vi "USBL_UA TRACKER for boat.vi"() -> ()   [LabVIEW 2017]
uses:
  <vilib>/Analysis/2dsp.llb/Decimate (single shot, DBL).vi
  <vilib>/DAQmx/read.llb/DAQmx Read (Analog 1D Wfm NChan NSamp).vi
  <vilib>/Analysis/3filter.llb/FIR Filter (DBL).vi
  <vilib>/DAQmx/create/channels.llb/DAQmx Create Channel (AI-Voltage-Basic).vi
  <vilib>/DAQmx/configure/timing.llb/DAQmx Timing (Sample Clock).vi
  <vilib>/DAQmx/miscellaneous.llb/DAQmx Fill In Error Info.vi
  <vilib>/DAQmx/create/channels.llb/DAQmx Create Channel (CO-Pulse Generation-Frequency).vi
  <vilib>/DAQmx/configure/timing.llb/DAQmx Timing (Implicit).vi
  <vilib>/Analysis/NI_AALBase.lvlib
  <vilib>/Analysis/NI_AALPro.lvlib
  <vilib>/Analysis/NI_AAL_SigProc.lvlib
  <resource>/objmgr/daqmx.rc
panel:
  out "숫자형 8":dbl=5.0
  out "Target code":dbl[](array[numeric])
  out "ThresholdMargin":dbl=10.0
  out "MovingAvrParm":dbl[](array[numeric])
  out "Coefficient_bit1":dbl[](array[numeric])
  out "Coefficient_bit0":dbl[](array[numeric])
  out "Decimation rate":i32=12
  out "Carrier signal":dbl[](array[numeric])
  out "숫자형 7":dbl=7.0
  out "숫자형 6":dbl=7.0
  out "숫자형 5":dbl=7.0
  in  "Number of pulse":i32=1000
  in  "Output terminal":tag="/Dev1/PFI12"
  in  "Frequency(Hz)":dbl=1.0 format="%.6f"
  in  "Cycle share":dbl=0.5 format="%.6f"
  in  "Counter":tag="Dev1/ctr0"
  out "Detect":bool
  in  "User number":i32=12
  out "숫자형 4":dbl=5.0
  out "숫자형 3":dbl=7.0
  out "숫자형 2":dbl=7.0
  out "숫자형":dbl=7.0
  in  "Start frequency(Hz)":dbl format="%#_6p"
  in  "Stop frequency(Hz)":dbl=4000.0 format="%#_6p"
  in  "Symbol length(sec)":dbl=0.128 format="%#_6p"
  in  "Number of sample":i32=38400
  in  "Sampling freuqncy(Hz)":dbl=192000.0 format="%#_6p"
  in  "Physical channel":tag="Dev4/ai0:7" caption="Physical Channel"
  in  "Device":tag="Dev4"
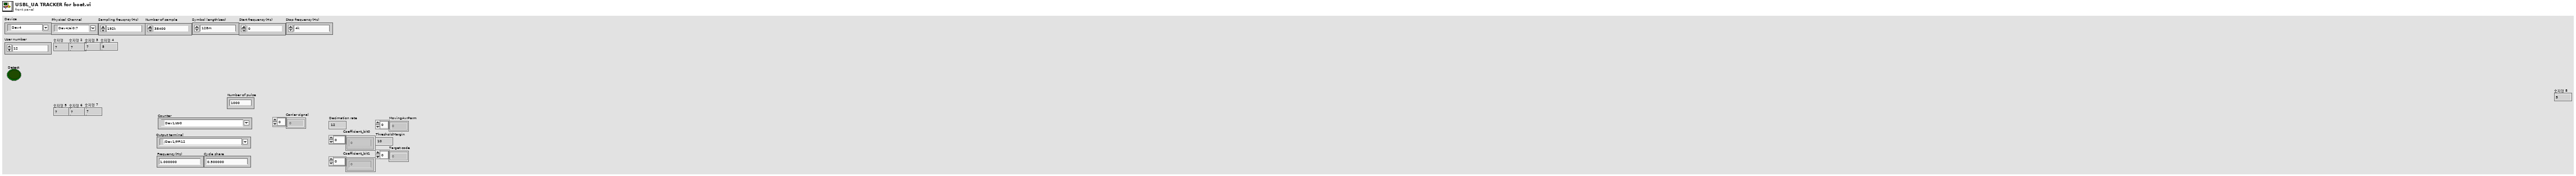
[diagram p1: front panel]
diagram:
  n1 = flat-sequence {
    tunnel: ["Number of sample"] -> w12
    tunnel: [w39] -> w11
    tunnel: ["Sampling freuqncy(Hz)"] -> w10
    tunnel: ["Physical channel"] -> w9
    tunnel: ["Device"] -> w8
    tunnel: [w35] -> w7
    tunnel: [w31] -> w6
    tunnel: [w30] -> w5
    tunnel: [w25] -> w4
    tunnel: [w21] -> w3
    tunnel: [w20] -> w2
    tunnel: [w13] -> w1
    tunnel: w12 -> [w59]
    tunnel: w11 -> [w58]
    tunnel: w10 -> [w57]
    tunnel: w9 -> [w56]
    tunnel: w8 -> [w55]
    tunnel: w7 -> [w54]
    tunnel: w6 -> [w53]
    tunnel: w5 -> [w52]
    tunnel: w4 -> [w49]
    tunnel: w3 -> [w47]
    tunnel: w2 -> [w46]
    tunnel: w1 -> [w43]
    frame #0 {
      w20 = 10.0 ("값")
      w22 = 160 ("차원 크기")
      w35 = 12 ("Divide by")
      w39 = 10123 items=["유한 샘플"=10178, "연속 샘플"=10123, "하드웨어 타이밍에 의한 단일 포인트"=12522] ("sample mode")
      # "Signal gen. (Counter)"
      # "Target code"
      # "EOF"
      # "SOF"
      # "Processing parameter"
      # "Freqeuncy 2"
      # "Freqeuncy 1"
      # "Symbol length"
      # "Moving average window size"
      # "Threshold Margin"
      # "DAQ device setting"
      # "Device"
      # "Physical channel"
      # "Sampling frequency"
      # "Sample mode"
      # "Number of samples per channel"
      n2 = To Double Precision Float(number=w35) -> (double precision float=w41:dbl)
      n3 = To Double Precision Float(number=w22) -> (double precision float=w24:dbl)
      n4 = Divide(x="Sampling freuqncy(Hz)", y=w41) -> (x/y=w29:dbl)
      n5 = Format Into String(format string="%04b" ("포맷 문자열"), "User number") -> (resulting string=w17:string)  [unwired: 2 in, 1 out]
      n6 = Reciprocal(x=w24) -> (1/x=w23:dbl)
      n7 = call "CodeConvert(SubVI).vi"("Code"=w17) -> ("Code_array"=w15:dbl[])
      n8 = Divide(x=30000.0, y="Sampling freuqncy(Hz)") -> (x/y=w33:dbl)
      n9 = Initialize Array(w23, w22) -> (w21:dbl[])
      "MovingAvrParm" <- w21
      n10 = call "ChirpSourceGen(SubVI).vi"("Frequency2(Hz)"="Stop frequency(Hz)", "Frequency1(Hz)"="Start frequency(Hz)", "Pulse length(sec)"="Symbol length(sec)", "Fs(Hz)"=w29) -> ("M.F. Tap(F2-1)"=w25:dbl[], "M.F. Tap(F1-2)"=w31:dbl[])  [unwired: 1 out]
      "Coefficient_bit0" <- w31
      "Coefficient_bit1" <- w25
      n11 = Insert Into Array(array=dbl[] [0.0, 1.0], new element #1=w15, new element #2=dbl[] [1.0, 0.0]) -> (w13:dbl[])  [unwired: 1 in]
      "Target code" <- w13
      n12 = call <vilib>:"Sine Wave.vi"("samples"="Number of sample", "amplitude"=5.0, "frequency"=w33) -> ("sine wave"=w30:dbl[])  [unwired: 2 in, 2 out]
      "Carrier signal" <- w30
      "Decimation rate" <- w35
      "ThresholdMargin" <- w20
    }
    frame #1 {
      n13 = flat-sequence {
        tunnel: w55 -> [w78]
        tunnel: [w79] -> w66
        tunnel: w56 -> [w77]
        tunnel: [w77] -> w65
        tunnel: w57 -> [w75]
        tunnel: [w75] -> w64
        tunnel: w59 -> [w74]
        tunnel: [w74] -> w63
        tunnel: w58 -> [w76]
        tunnel: [w76] -> w62
        tunnel: [w72] -> w61
        tunnel: [w73] -> w60
        tunnel: w54 -> [w73]
        tunnel: w53 -> [w72]
        tunnel: w52 -> [w71]
        tunnel: [w71] -> w51
        tunnel: [w70] -> w50
        tunnel: w49 -> [w70]
        tunnel: [w69] -> w48
        tunnel: w47 -> [w69]
        tunnel: w46 -> [w68]
        tunnel: [w68] -> w45
        tunnel: [w67] -> w44
        tunnel: w43 -> [w67]
        tunnel: w66 -> [w123]
        tunnel: w65 -> [w122]
        tunnel: w64 -> [w121]
        tunnel: w63 -> [w119]
        tunnel: w62 -> [w120]
        tunnel: w61 -> [w108]
        tunnel: w60 -> [w96]
        tunnel: w51 -> [w97]
        tunnel: w50 -> [w81]
        tunnel: w48 -> [w88]
        tunnel: w45 -> [w87]
        tunnel: w44 -> [w82]
        tunnel: [w430] -> w42
        tunnel: w42 -> [w523]
        frame #0 {
          n14 = call <vilib>:"DAQmx Reset Device.vi"("device in"=w78) -> ("error out"=w79:errorcluster)  [unwired: 1 in, 13 out]
        }
        frame #1 {
          w80 = dbl[] [-1.0, -1.0, -1.0, -1.0, -1.0, -1.0, -1.0, -1.0]
          w94 = "Proc1" ("이름(이름없음)")
          w95 = "Proc0" ("이름(이름없음)")
          w93 = dbl[][] []
          w109 = "SIG0" ("이름(이름없음)")
          w116 = waveform(dbl) {"t0"=timestamp(0 s since 1904-01-01), "dt"=1.0, "Y"=[]} ("Waveform")
          w99 = "SIG1" ("이름(이름없음)")
          # "Target code"
          # "[Post processing]  1. Queue get : Proc0, Proc1 / 2. Threshold estimation with moving average / 3. Peak and valley detection / 4. Demodulation"
          # "[Signal processing]\n1. Queue get : SIG0\n2. Data type converting : Waveform (DBL) --> Array (DBL)\n3. DDC (Digital to Digital Convering)\n  - DSB modulation : Multiply carrier signal (30kHz)\n  - Decimate : 192kHz sample rate --> 16kHz sample rate\n4. Cross-correlation with down-chirp (4k ~ 0Hz)\n5. Envelope detection (Hilbert transform) & square\n6. Queue put : Proc1"
          # "[Signal processing]\n1. Queue get : SIG0\n2. Data type converting : Waveform (DBL) --> Array (DBL)\n3. DDC (Digital to Digital Convering)\n  - DSB modulation : Multiply carrier signal (30kHz)\n  - Decimate : 192kHz sample rate --> 16kHz sample rate\n4. Cross-correlation with up-chirp (0 ~ 4kHz)\n5. Envelope detection (Hilbert transform) & square\n6. Queue put : Proc0"
          # "[Data Acquistion (ADC)]\n1. Device reset\n2. Creat channel\n3, Set sample clock\n  - Sampling frequency : 192kHz\n  - Number of sample (Chunk size) : 38400\n4. Start task\n5. Data read\n6. Queue put : SIG0, SIG1\n  - Queue data type : Waveform (DBL)"
          # "Moving average prameter based on FIR filter calculation"
          # "Coefficient for bit 1 : Down-chirp"
          # "Coefficient for bit 0 : Up-chirp"
          # "Decimation rate"
          # "Carrier signal"
          n15 = call-poly <vilib>:"DAQmx Create Virtual Channel.vi"("physical channels"=w122, "error in"=w123) -> ("task out"=w125:refnum<k21>, "error out"=w124:errorcluster)  [unwired: 7 in, 5 out]
          n16 = call-poly <vilib>:"DAQmx Timing.vi"("task/channels in"=w125, "sample mode"=w120, "samples per channel"=w119, "rate"=w121, "error in"=w124) -> ("task out"=w126:refnum<k21>, "error out"=w127:errorcluster)  [unwired: 2 in, 7 out]
          n17 = call <vilib>:"DAQmx Start Task.vi"("task/channels in"=w126, "error in"=w127) -> ("task out"=w128:refnum<k21>, "error out"=w129:errorcluster)  [unwired: 12 in]
          n18 = Build Array(w116, w116, w116, w116, w116, w116, w116, w116) -> (w98:waveform(dbl)[])
          n19 = Obtain Queue(name (unnamed)=w99, element data type=w98) -> (queue out=w118:refnum<queue>, error out=w117:errorcluster)  [unwired: 3 in, 1 out]
          n20 = Obtain Queue(name (unnamed)=w109, element data type=w98) -> (queue out=w115:refnum<queue>, error out=w114:errorcluster)  [unwired: 3 in, 1 out]
          n21 = while {
            tunnel: w128 -> [w429]
            tunnel: w129 -> [w428]
            tunnel: [w427] -> w132
            tunnel: [w426] -> w133
            tunnel: w119 -> [w425]
            tunnel: w118 -> [w424]
            tunnel: w117 -> [w423]
            tunnel: w115 -> [w422]
            tunnel: w114 -> [w421]
            i -> [w419]
            stop <- w418 stop-if-true
            n22 = call-poly <vilib>:"DAQmx Read.vi"("task/channels in"=w429, "number of samples per channel"=w425, "error in"=w428) -> ("task out"=w427:refnum<k21>, "data"=w420:waveform(dbl)[], "error out"=w426:errorcluster)  [unwired: 10 out]
            n23 = Enqueue Element(queue=w422, element=w420, error in (no error)=w421) -> ()  [unwired: 1 in, 3 out]
            n24 = Enqueue Element(queue=w424, element=w420, error in (no error)=w423) -> ()  [unwired: 1 in, 3 out]
            n25 = local read "Detect"() -> (w418:bool)
            "숫자형" <- w419
          }
          n26 = call <vilib>:"DAQmx Stop Task.vi"("task/channels in"=w132, "error in"=w133) -> ("task out"=w131:refnum<k21>, "error out"=w130:errorcluster)  [unwired: 12 out]
          n27 = call <vilib>:"DAQmx Clear Task.vi"("task in"=w131, "error in"=w130) -> ()  [unwired: 14 out]
          n28 = Obtain Queue(name (unnamed)=w95, element data type=w93) -> (queue out=w113:refnum<queue>, error out=w112:errorcluster)  [unwired: 3 in, 1 out]
          n29 = Obtain Queue(name (unnamed)=w109, element data type=w98) -> (queue out=w111:refnum<queue>, error out=w110:errorcluster)  [unwired: 3 in, 1 out]
          n30 = while {
            tunnel: w111 -> [w417]
            tunnel: w110 -> [w416]
            tunnel: w113 -> [w415]
            tunnel: w112 -> [w414]
            tunnel: [w413] -> w107
            tunnel: [w412] -> w106
            tunnel: w97 -> [w352]
            tunnel: w96 -> [w351]
            tunnel: w108 -> [w350]
            i -> [w348]
            stop <- w347 stop-if-true
            w362 = TRUE ("averaging")
            w411 = TRUE ("init/cont (init:F)")
            n31 = Dequeue Element(queue=w417, error in (no error)=w416) -> (queue out=w413:refnum<queue>, element=w353:waveform(dbl)[], error out=w412:errorcluster)  [unwired: 2 out]
            n32 = Index Array(array=w353) -> (element #1=w410:waveform(dbl), element #2=w409:waveform(dbl), element #3=w408:waveform(dbl), element #4=w407:waveform(dbl), element #5=w406:waveform(dbl), element #6=w405:waveform(dbl), element #7=w404:waveform(dbl), element #8=w403:waveform(dbl))  [unwired: 8 in]
            n33 = Unbundle By Name(w410) -> ("Y"=w402:dbl[])
            n34 = Unbundle By Name(w409) -> ("Y"=w401:dbl[])
            n35 = Unbundle By Name(w408) -> ("Y"=w400:dbl[])
            n36 = Unbundle By Name(w407) -> ("Y"=w399:dbl[])
            n37 = Unbundle By Name(w406) -> ("Y"=w398:dbl[])
            n38 = Unbundle By Name(w405) -> ("Y"=w397:dbl[])
            n39 = Unbundle By Name(w404) -> ("Y"=w396:dbl[])
            n40 = Unbundle By Name(w403) -> ("Y"=w395:dbl[])
            n41 = Multiply(x=w402, y=w352) -> (x*y=w377:dbl[])
            n42 = Multiply(x=w401, y=w352) -> (x*y=w376:dbl[])
            n43 = Multiply(x=w400, y=w352) -> (x*y=w375:dbl[])
            n44 = Multiply(x=w399, y=w352) -> (x*y=w374:dbl[])
            n45 = Multiply(x=w398, y=w352) -> (x*y=w373:dbl[])
            n46 = Multiply(x=w397, y=w352) -> (x*y=w372:dbl[])
            n47 = Multiply(x=w396, y=w352) -> (x*y=w371:dbl[])
            n48 = Multiply(x=w395, y=w352) -> (x*y=w370:dbl[])
            n49 = call-poly <vilib>:"Decimate (single shot).vi"("averaging"=w362, "decimating factor"=w351, "X"=w372) -> ("Decimated Array"=w365:dbl[])  [unwired: 7 in, 1 out]
            n50 = call-poly <vilib>:"Decimate (single shot).vi"("averaging"=w362, "decimating factor"=w351, "X"=w370) -> ("Decimated Array"=w363:dbl[])  [unwired: 7 in, 1 out]
            n51 = call-poly <vilib>:"Decimate (single shot).vi"("averaging"=w362, "decimating factor"=w351, "X"=w376) -> ("Decimated Array"=w369:dbl[])  [unwired: 7 in, 1 out]
            n52 = call-poly <vilib>:"Decimate (single shot).vi"("averaging"=w362, "decimating factor"=w351, "X"=w374) -> ("Decimated Array"=w367:dbl[])  [unwired: 7 in, 1 out]
            n53 = call-poly <vilib>:"Decimate (single shot).vi"("averaging"=w362, "decimating factor"=w351, "X"=w373) -> ("Decimated Array"=w366:dbl[])  [unwired: 7 in, 1 out]
            n54 = call-poly <vilib>:"Decimate (single shot).vi"("averaging"=w362, "decimating factor"=w351, "X"=w371) -> ("Decimated Array"=w364:dbl[])  [unwired: 7 in, 1 out]
            n55 = call-poly <vilib>:"Decimate (single shot).vi"("averaging"=w362, "decimating factor"=w351, "X"=w377) -> ("Decimated Array"=w378:dbl[])  [unwired: 7 in, 1 out]
            n56 = call-poly <vilib>:"Decimate (single shot).vi"("averaging"=w362, "decimating factor"=w351, "X"=w375) -> ("Decimated Array"=w368:dbl[])  [unwired: 7 in, 1 out]
            n57 = call-poly <vilib>:"FIR Filter.vi"("init/cont (init:F)"=w411, "FIR Coefficients"=w350, "X"=w378) -> ("Filtered X"=w394:dbl[])  [unwired: 1 in, 1 out]
            n58 = call-poly <vilib>:"FIR Filter.vi"("init/cont (init:F)"=w411, "FIR Coefficients"=w350, "X"=w369) -> ("Filtered X"=w393:dbl[])  [unwired: 1 in, 1 out]
            n59 = call-poly <vilib>:"FIR Filter.vi"("init/cont (init:F)"=w411, "FIR Coefficients"=w350, "X"=w368) -> ("Filtered X"=w392:dbl[])  [unwired: 1 in, 1 out]
            n60 = call-poly <vilib>:"FIR Filter.vi"("init/cont (init:F)"=w411, "FIR Coefficients"=w350, "X"=w367) -> ("Filtered X"=w391:dbl[])  [unwired: 1 in, 1 out]
            n61 = call-poly <vilib>:"FIR Filter.vi"("init/cont (init:F)"=w411, "FIR Coefficients"=w350, "X"=w366) -> ("Filtered X"=w390:dbl[])  [unwired: 1 in, 1 out]
            n62 = call-poly <vilib>:"FIR Filter.vi"("init/cont (init:F)"=w411, "FIR Coefficients"=w350, "X"=w365) -> ("Filtered X"=w389:dbl[])  [unwired: 1 in, 1 out]
            n63 = call-poly <vilib>:"FIR Filter.vi"("init/cont (init:F)"=w411, "FIR Coefficients"=w350, "X"=w364) -> ("Filtered X"=w388:dbl[])  [unwired: 1 in, 1 out]
            n64 = call-poly <vilib>:"FIR Filter.vi"("init/cont (init:F)"=w411, "FIR Coefficients"=w350, "X"=w363) -> ("Filtered X"=w387:dbl[])  [unwired: 1 in, 1 out]
            n65 = call "Envelope(SubVI).vi"("x"=w394) -> ("Y"=w386:dbl[])
            n66 = call "Envelope(SubVI).vi"("x"=w393) -> ("Y"=w385:dbl[])
            n67 = call "Envelope(SubVI).vi"("x"=w392) -> ("Y"=w384:dbl[])
            n68 = call "Envelope(SubVI).vi"("x"=w391) -> ("Y"=w383:dbl[])
            n69 = call "Envelope(SubVI).vi"("x"=w390) -> ("Y"=w382:dbl[])
            n70 = call "Envelope(SubVI).vi"("x"=w389) -> ("Y"=w381:dbl[])
            n71 = call "Envelope(SubVI).vi"("x"=w388) -> ("Y"=w380:dbl[])
            n72 = call "Envelope(SubVI).vi"("x"=w387) -> ("Y"=w379:dbl[])
            n73 = Square(x=w386) -> (x^2=w361:dbl[])
            n74 = Square(x=w385) -> (x^2=w360:dbl[])
            n75 = Square(x=w384) -> (x^2=w359:dbl[])
            n76 = Square(x=w383) -> (x^2=w358:dbl[])
            n77 = Square(x=w382) -> (x^2=w357:dbl[])
            n78 = Square(x=w381) -> (x^2=w356:dbl[])
            n79 = Square(x=w380) -> (x^2=w355:dbl[])
            n80 = Square(x=w379) -> (x^2=w354:dbl[])
            n81 = local read "Detect"() -> (w347:bool)
            n82 = Build Array(w361, w360, w359, w358, w357, w356, w355, w354) -> (w349:dbl[][])
            n83 = Enqueue Element(queue=w415, element=w349, error in (no error)=w414) -> ()  [unwired: 1 in, 3 out]
            "숫자형 2" <- w348
          }
          n84 = Release Queue(queue=w107, error in (no error)=w106) -> ()  [unwired: 1 in, 3 out]
          n85 = Obtain Queue(name (unnamed)=w94, element data type=w93) -> (queue out=w105:refnum<queue>, error out=w104:errorcluster)  [unwired: 3 in, 1 out]
          n86 = Obtain Queue(name (unnamed)=w99, element data type=w98) -> (queue out=w103:refnum<queue>, error out=w102:errorcluster)  [unwired: 3 in, 1 out]
          n87 = while {
            tunnel: w103 -> [w346]
            tunnel: w102 -> [w345]
            tunnel: w105 -> [w344]
            tunnel: w104 -> [w343]
            tunnel: [w342] -> w101
            tunnel: [w341] -> w100
            tunnel: w97 -> [w281]
            tunnel: w96 -> [w280]
            tunnel: w81 -> [w279]
            i -> [w277]
            stop <- w276 stop-if-true
            w291 = TRUE ("averaging")
            w340 = TRUE ("init/cont (init:F)")
            n88 = Dequeue Element(queue=w346, error in (no error)=w345) -> (queue out=w342:refnum<queue>, element=w282:waveform(dbl)[], error out=w341:errorcluster)  [unwired: 2 out]
            n89 = Index Array(array=w282) -> (element #1=w339:waveform(dbl), element #2=w338:waveform(dbl), element #3=w337:waveform(dbl), element #4=w336:waveform(dbl), element #5=w335:waveform(dbl), element #6=w334:waveform(dbl), element #7=w333:waveform(dbl), element #8=w332:waveform(dbl))  [unwired: 8 in]
            n90 = Unbundle By Name(w339) -> ("Y"=w331:dbl[])
            n91 = Unbundle By Name(w338) -> ("Y"=w330:dbl[])
            n92 = Unbundle By Name(w337) -> ("Y"=w329:dbl[])
            n93 = Unbundle By Name(w336) -> ("Y"=w328:dbl[])
            n94 = Unbundle By Name(w335) -> ("Y"=w327:dbl[])
            n95 = Unbundle By Name(w334) -> ("Y"=w326:dbl[])
            n96 = Unbundle By Name(w333) -> ("Y"=w325:dbl[])
            n97 = Unbundle By Name(w332) -> ("Y"=w324:dbl[])
            n98 = Multiply(x=w331, y=w281) -> (x*y=w306:dbl[])
            n99 = Multiply(x=w330, y=w281) -> (x*y=w305:dbl[])
            n100 = Multiply(x=w329, y=w281) -> (x*y=w304:dbl[])
            n101 = Multiply(x=w328, y=w281) -> (x*y=w303:dbl[])
            n102 = Multiply(x=w327, y=w281) -> (x*y=w302:dbl[])
            n103 = Multiply(x=w326, y=w281) -> (x*y=w301:dbl[])
            n104 = Multiply(x=w325, y=w281) -> (x*y=w300:dbl[])
            n105 = Multiply(x=w324, y=w281) -> (x*y=w299:dbl[])
            n106 = call-poly <vilib>:"Decimate (single shot).vi"("averaging"=w291, "decimating factor"=w280, "X"=w301) -> ("Decimated Array"=w294:dbl[])  [unwired: 7 in, 1 out]
            n107 = call-poly <vilib>:"Decimate (single shot).vi"("averaging"=w291, "decimating factor"=w280, "X"=w299) -> ("Decimated Array"=w292:dbl[])  [unwired: 7 in, 1 out]
            n108 = call-poly <vilib>:"Decimate (single shot).vi"("averaging"=w291, "decimating factor"=w280, "X"=w305) -> ("Decimated Array"=w298:dbl[])  [unwired: 7 in, 1 out]
            n109 = call-poly <vilib>:"Decimate (single shot).vi"("averaging"=w291, "decimating factor"=w280, "X"=w303) -> ("Decimated Array"=w296:dbl[])  [unwired: 7 in, 1 out]
            n110 = call-poly <vilib>:"Decimate (single shot).vi"("averaging"=w291, "decimating factor"=w280, "X"=w302) -> ("Decimated Array"=w295:dbl[])  [unwired: 7 in, 1 out]
            n111 = call-poly <vilib>:"Decimate (single shot).vi"("averaging"=w291, "decimating factor"=w280, "X"=w300) -> ("Decimated Array"=w293:dbl[])  [unwired: 7 in, 1 out]
            n112 = call-poly <vilib>:"Decimate (single shot).vi"("averaging"=w291, "decimating factor"=w280, "X"=w306) -> ("Decimated Array"=w307:dbl[])  [unwired: 7 in, 1 out]
            n113 = call-poly <vilib>:"Decimate (single shot).vi"("averaging"=w291, "decimating factor"=w280, "X"=w304) -> ("Decimated Array"=w297:dbl[])  [unwired: 7 in, 1 out]
            n114 = call-poly <vilib>:"FIR Filter.vi"("init/cont (init:F)"=w340, "FIR Coefficients"=w279, "X"=w307) -> ("Filtered X"=w323:dbl[])  [unwired: 1 in, 1 out]
            n115 = call-poly <vilib>:"FIR Filter.vi"("init/cont (init:F)"=w340, "FIR Coefficients"=w279, "X"=w298) -> ("Filtered X"=w322:dbl[])  [unwired: 1 in, 1 out]
            n116 = call-poly <vilib>:"FIR Filter.vi"("init/cont (init:F)"=w340, "FIR Coefficients"=w279, "X"=w297) -> ("Filtered X"=w321:dbl[])  [unwired: 1 in, 1 out]
            n117 = call-poly <vilib>:"FIR Filter.vi"("init/cont (init:F)"=w340, "FIR Coefficients"=w279, "X"=w296) -> ("Filtered X"=w320:dbl[])  [unwired: 1 in, 1 out]
            n118 = call-poly <vilib>:"FIR Filter.vi"("init/cont (init:F)"=w340, "FIR Coefficients"=w279, "X"=w295) -> ("Filtered X"=w319:dbl[])  [unwired: 1 in, 1 out]
            n119 = call-poly <vilib>:"FIR Filter.vi"("init/cont (init:F)"=w340, "FIR Coefficients"=w279, "X"=w294) -> ("Filtered X"=w318:dbl[])  [unwired: 1 in, 1 out]
            n120 = call-poly <vilib>:"FIR Filter.vi"("init/cont (init:F)"=w340, "FIR Coefficients"=w279, "X"=w293) -> ("Filtered X"=w317:dbl[])  [unwired: 1 in, 1 out]
            n121 = call-poly <vilib>:"FIR Filter.vi"("init/cont (init:F)"=w340, "FIR Coefficients"=w279, "X"=w292) -> ("Filtered X"=w316:dbl[])  [unwired: 1 in, 1 out]
            n122 = call "Envelope(SubVI).vi"("x"=w323) -> ("Y"=w315:dbl[])
            n123 = call "Envelope(SubVI).vi"("x"=w322) -> ("Y"=w314:dbl[])
            n124 = call "Envelope(SubVI).vi"("x"=w321) -> ("Y"=w313:dbl[])
            n125 = call "Envelope(SubVI).vi"("x"=w320) -> ("Y"=w312:dbl[])
            n126 = call "Envelope(SubVI).vi"("x"=w319) -> ("Y"=w311:dbl[])
            n127 = call "Envelope(SubVI).vi"("x"=w318) -> ("Y"=w310:dbl[])
            n128 = call "Envelope(SubVI).vi"("x"=w317) -> ("Y"=w309:dbl[])
            n129 = call "Envelope(SubVI).vi"("x"=w316) -> ("Y"=w308:dbl[])
            n130 = Square(x=w315) -> (x^2=w290:dbl[])
            n131 = Square(x=w314) -> (x^2=w289:dbl[])
            n132 = Square(x=w313) -> (x^2=w288:dbl[])
            n133 = Square(x=w312) -> (x^2=w287:dbl[])
            n134 = Square(x=w311) -> (x^2=w286:dbl[])
            n135 = Square(x=w310) -> (x^2=w285:dbl[])
            n136 = Square(x=w309) -> (x^2=w284:dbl[])
            n137 = Square(x=w308) -> (x^2=w283:dbl[])
            n138 = local read "Detect"() -> (w276:bool)
            n139 = Build Array(w290, w289, w288, w287, w286, w285, w284, w283) -> (w278:dbl[][])
            n140 = Enqueue Element(queue=w344, element=w278, error in (no error)=w343) -> ()  [unwired: 1 in, 3 out]
            "숫자형 3" <- w277
          }
          n141 = Release Queue(queue=w101, error in (no error)=w100) -> ()  [unwired: 1 in, 3 out]
          n142 = Obtain Queue(name (unnamed)=w95, element data type=w93) -> (queue out=w92:refnum<queue>, error out=w91:errorcluster)  [unwired: 3 in, 1 out]
          n143 = Obtain Queue(name (unnamed)=w94, element data type=w93) -> (queue out=w90:refnum<queue>, error out=w89:errorcluster)  [unwired: 3 in, 1 out]
          n144 = while {
            tunnel: w92 -> [w275]
            tunnel: w91 -> [w274]
            tunnel: w90 -> [w273]
            tunnel: w89 -> [w272]
            tunnel: w88 -> [w270]
            tunnel: w87 -> [w234]
            tunnel: [w182] -> w86
            tunnel: [w181] -> w85
            tunnel: [w180] -> w84
            tunnel: [w179] -> w83
            tunnel: w82 -> [w178]
            shift-right: [w141] -> _
            shift-left: w80 -> [w157]
            shift-right: [w140] -> _
            shift-left: w80 -> [w156]
            shift-right: [w139] -> _
            shift-left: w80 -> [w155]
            shift-right: [w138] -> _
            shift-left: w80 -> [w154]
            shift-right: [w137] -> _
            shift-left: w80 -> [w153]
            shift-right: [w136] -> _
            shift-left: w80 -> [w152]
            shift-right: [w135] -> _
            shift-left: w80 -> [w151]
            shift-right: [w134] -> _
            shift-left: w80 -> [w150]
            i -> [w166]
            stop <- w167 stop-if-true
            w259 = enum32{"Peaks", "Valleys"}."Valleys" ("peaks/valleys")
            w260 = enum32{"Peaks", "Valleys"}."Peaks" ("peaks/valleys")
            w258 = 5 ("width")
            w269 = TRUE ("init/cont (init:F)")
            n145 = Dequeue Element(queue=w275, error in (no error)=w274) -> (queue out=w182:refnum<queue>, element=w216:dbl[][], error out=w181:errorcluster)  [unwired: 2 out]
            n146 = Dequeue Element(queue=w273, error in (no error)=w272) -> (queue out=w180:refnum<queue>, element=w215:dbl[][], error out=w179:errorcluster)  [unwired: 2 out]
            n147 = Subtract(x=w216, y=w215) -> (x-y=w271:dbl[][])
            n148 = Index Array(array=w271) -> (element #1=w257:dbl[], element #2=w256:dbl[], element #3=w255:dbl[], element #4=w254:dbl[], element #5=w253:dbl[], element #6=w252:dbl[], element #7=w251:dbl[], element #8=w219:dbl[])  [unwired: 16 in]
            n149 = call-poly <vilib>:"FIR Filter.vi"("init/cont (init:F)"=w269, "FIR Coefficients"=w270, "X"=w257) -> ("Filtered X"=w268:dbl[])  [unwired: 1 in, 1 out]
            n150 = call-poly <vilib>:"FIR Filter.vi"("init/cont (init:F)"=w269, "FIR Coefficients"=w270, "X"=w256) -> ("Filtered X"=w267:dbl[])  [unwired: 1 in, 1 out]
            n151 = call-poly <vilib>:"FIR Filter.vi"("init/cont (init:F)"=w269, "FIR Coefficients"=w270, "X"=w255) -> ("Filtered X"=w266:dbl[])  [unwired: 1 in, 1 out]
            n152 = call-poly <vilib>:"FIR Filter.vi"("init/cont (init:F)"=w269, "FIR Coefficients"=w270, "X"=w254) -> ("Filtered X"=w265:dbl[])  [unwired: 1 in, 1 out]
            n153 = call-poly <vilib>:"FIR Filter.vi"("init/cont (init:F)"=w269, "FIR Coefficients"=w270, "X"=w253) -> ("Filtered X"=w264:dbl[])  [unwired: 1 in, 1 out]
            n154 = call-poly <vilib>:"FIR Filter.vi"("init/cont (init:F)"=w269, "FIR Coefficients"=w270, "X"=w252) -> ("Filtered X"=w263:dbl[])  [unwired: 1 in, 1 out]
            n155 = call-poly <vilib>:"FIR Filter.vi"("init/cont (init:F)"=w269, "FIR Coefficients"=w270, "X"=w251) -> ("Filtered X"=w262:dbl[])  [unwired: 1 in, 1 out]
            n156 = call-poly <vilib>:"FIR Filter.vi"("init/cont (init:F)"=w269, "FIR Coefficients"=w270, "X"=w219) -> ("Filtered X"=w261:dbl[])  [unwired: 1 in, 1 out]
            n157 = Array Max & Min(array=w268) -> (max value=w250:dbl, min value=w249:dbl)  [unwired: 2 out]
            n158 = Array Max & Min(array=w267) -> (max value=w248:dbl, min value=w247:dbl)  [unwired: 2 out]
            n159 = Array Max & Min(array=w266) -> (max value=w246:dbl, min value=w245:dbl)  [unwired: 2 out]
            n160 = Array Max & Min(array=w265) -> (max value=w244:dbl, min value=w243:dbl)  [unwired: 2 out]
            n161 = Array Max & Min(array=w264) -> (max value=w242:dbl, min value=w241:dbl)  [unwired: 2 out]
            n162 = Array Max & Min(array=w263) -> (max value=w240:dbl, min value=w239:dbl)  [unwired: 2 out]
            n163 = Array Max & Min(array=w262) -> (max value=w238:dbl, min value=w237:dbl)  [unwired: 2 out]
            n164 = Array Max & Min(array=w261) -> (max value=w236:dbl, min value=w235:dbl)  [unwired: 2 out]
            n165 = call "ThresholdEstimation(SubVI).vi"("Margin"=w234, "최소값"=w247, "최대값"=w248) -> ("N.Th"=w221:dbl, "P.Th"=w232:dbl)
            n166 = call "ThresholdEstimation(SubVI).vi"("Margin"=w234, "최소값"=w245, "최대값"=w246) -> ("N.Th"=w222:dbl, "P.Th"=w231:dbl)
            n167 = call "ThresholdEstimation(SubVI).vi"("Margin"=w234, "최소값"=w243, "최대값"=w244) -> ("N.Th"=w223:dbl, "P.Th"=w230:dbl)
            n168 = call "ThresholdEstimation(SubVI).vi"("Margin"=w234, "최소값"=w241, "최대값"=w242) -> ("N.Th"=w224:dbl, "P.Th"=w229:dbl)
            n169 = call "ThresholdEstimation(SubVI).vi"("Margin"=w234, "최소값"=w249, "최대값"=w250) -> ("N.Th"=w220:dbl, "P.Th"=w233:dbl)
            n170 = call "ThresholdEstimation(SubVI).vi"("Margin"=w234, "최소값"=w239, "최대값"=w240) -> ("N.Th"=w225:dbl, "P.Th"=w228:dbl)
            n171 = call "ThresholdEstimation(SubVI).vi"("Margin"=w234, "최소값"=w237, "최대값"=w238) -> ("N.Th"=w226:dbl, "P.Th"=w227:dbl)
            n172 = call "ThresholdEstimation(SubVI).vi"("Margin"=w234, "최소값"=w235, "최대값"=w236) -> ("N.Th"=w218:dbl, "P.Th"=w217:dbl)
            n173 = call <vilib>:"Peak Detector.vi"("peaks/valleys"=w260, "width"=w258, "threshold"=w233, "X"=w257) -> ("Locations"=w191:dbl[], "# found"=w207:i32)  [unwired: 3 in, 3 out]
            n174 = call <vilib>:"Peak Detector.vi"("peaks/valleys"=w260, "width"=w258, "threshold"=w232, "X"=w256) -> ("Locations"=w192:dbl[], "# found"=w208:i32)  [unwired: 3 in, 3 out]
            n175 = call <vilib>:"Peak Detector.vi"("peaks/valleys"=w260, "width"=w258, "threshold"=w231, "X"=w255) -> ("Locations"=w193:dbl[], "# found"=w209:i32)  [unwired: 3 in, 3 out]
            n176 = call <vilib>:"Peak Detector.vi"("peaks/valleys"=w260, "width"=w258, "threshold"=w230, "X"=w254) -> ("Locations"=w194:dbl[], "# found"=w210:i32)  [unwired: 3 in, 3 out]
            n177 = call <vilib>:"Peak Detector.vi"("peaks/valleys"=w260, "width"=w258, "threshold"=w229, "X"=w253) -> ("Locations"=w195:dbl[], "# found"=w211:i32)  [unwired: 3 in, 3 out]
            n178 = call <vilib>:"Peak Detector.vi"("peaks/valleys"=w260, "width"=w258, "threshold"=w228, "X"=w252) -> ("Locations"=w196:dbl[], "# found"=w212:i32)  [unwired: 3 in, 3 out]
            n179 = call <vilib>:"Peak Detector.vi"("peaks/valleys"=w260, "width"=w258, "threshold"=w227, "X"=w251) -> ("Locations"=w197:dbl[], "# found"=w213:i32)  [unwired: 3 in, 3 out]
            n180 = call <vilib>:"Peak Detector.vi"("peaks/valleys"=w260, "width"=w258, "threshold"=w217, "X"=w219) -> ("Locations"=w198:dbl[], "# found"=w214:i32)  [unwired: 3 in, 3 out]
            n181 = call <vilib>:"Peak Detector.vi"("peaks/valleys"=w259, "width"=w258, "threshold"=w220, "X"=w257) -> ("Locations"=w190:dbl[], "# found"=w206:i32)  [unwired: 3 in, 3 out]
            n182 = call <vilib>:"Peak Detector.vi"("peaks/valleys"=w259, "width"=w258, "threshold"=w221, "X"=w256) -> ("Locations"=w189:dbl[], "# found"=w205:i32)  [unwired: 3 in, 3 out]
            n183 = call <vilib>:"Peak Detector.vi"("peaks/valleys"=w259, "width"=w258, "threshold"=w222, "X"=w255) -> ("Locations"=w188:dbl[], "# found"=w204:i32)  [unwired: 3 in, 3 out]
            n184 = call <vilib>:"Peak Detector.vi"("peaks/valleys"=w259, "width"=w258, "threshold"=w223, "X"=w254) -> ("Locations"=w187:dbl[], "# found"=w203:i32)  [unwired: 3 in, 3 out]
            n185 = call <vilib>:"Peak Detector.vi"("peaks/valleys"=w259, "width"=w258, "threshold"=w224, "X"=w253) -> ("Locations"=w186:dbl[], "# found"=w202:i32)  [unwired: 3 in, 3 out]
            n186 = call <vilib>:"Peak Detector.vi"("peaks/valleys"=w259, "width"=w258, "threshold"=w225, "X"=w252) -> ("Locations"=w185:dbl[], "# found"=w201:i32)  [unwired: 3 in, 3 out]
            n187 = call <vilib>:"Peak Detector.vi"("peaks/valleys"=w259, "width"=w258, "threshold"=w226, "X"=w251) -> ("Locations"=w184:dbl[], "# found"=w200:i32)  [unwired: 3 in, 3 out]
            n188 = call <vilib>:"Peak Detector.vi"("peaks/valleys"=w259, "width"=w258, "threshold"=w218, "X"=w219) -> ("Locations"=w183:dbl[], "# found"=w199:i32)  [unwired: 3 in, 3 out]
            n189 = call "Decision(SubVI).vi"("L_ind0"=w207, "L_ind1"=w206, "Peak_ind0"=w191, "Peak_ind1"=w190) -> ("L_sum"=w149:i32, "Bits"=w165:dbl[])  [unwired: 2 in]
            n190 = call "Decision(SubVI).vi"("L_ind0"=w208, "L_ind1"=w205, "Peak_ind0"=w192, "Peak_ind1"=w189) -> ("L_sum"=w148:i32, "Bits"=w164:dbl[])  [unwired: 2 in]
            n191 = call "Decision(SubVI).vi"("L_ind0"=w209, "L_ind1"=w204, "Peak_ind0"=w193, "Peak_ind1"=w188) -> ("L_sum"=w147:i32, "Bits"=w163:dbl[])  [unwired: 2 in]
            n192 = call "Decision(SubVI).vi"("L_ind0"=w210, "L_ind1"=w203, "Peak_ind0"=w194, "Peak_ind1"=w187) -> ("L_sum"=w146:i32, "Bits"=w162:dbl[])  [unwired: 2 in]
            n193 = call "Decision(SubVI).vi"("L_ind0"=w211, "L_ind1"=w202, "Peak_ind0"=w195, "Peak_ind1"=w186) -> ("L_sum"=w145:i32, "Bits"=w161:dbl[])  [unwired: 2 in]
            n194 = call "Decision(SubVI).vi"("L_ind0"=w212, "L_ind1"=w201, "Peak_ind0"=w196, "Peak_ind1"=w185) -> ("L_sum"=w144:i32, "Bits"=w160:dbl[])  [unwired: 2 in]
            n195 = call "Decision(SubVI).vi"("L_ind0"=w213, "L_ind1"=w200, "Peak_ind0"=w197, "Peak_ind1"=w184) -> ("L_sum"=w143:i32, "Bits"=w159:dbl[])  [unwired: 2 in]
            n196 = call "Decision(SubVI).vi"("L_ind0"=w214, "L_ind1"=w199, "Peak_ind0"=w198, "Peak_ind1"=w183) -> ("L_sum"=w142:i32, "Bits"=w158:dbl[])  [unwired: 2 in]
            n197 = call "DataBuffer(SubVI).vi"("Bits"=w165, "Buffer"=w157) -> ("Data"=w141:dbl[])  [unwired: 2 in]
            n198 = call "DataBuffer(SubVI).vi"("Bits"=w164, "Buffer"=w156) -> ("Data"=w140:dbl[])  [unwired: 2 in]
            n199 = call "DataBuffer(SubVI).vi"("Bits"=w163, "Buffer"=w155) -> ("Data"=w139:dbl[])  [unwired: 2 in]
            n200 = call "DataBuffer(SubVI).vi"("Bits"=w162, "Buffer"=w154) -> ("Data"=w138:dbl[])  [unwired: 2 in]
            n201 = call "DataBuffer(SubVI).vi"("Bits"=w161, "Buffer"=w153) -> ("Data"=w137:dbl[])  [unwired: 2 in]
            n202 = call "DataBuffer(SubVI).vi"("Bits"=w160, "Buffer"=w152) -> ("Data"=w136:dbl[])  [unwired: 2 in]
            n203 = call "DataBuffer(SubVI).vi"("Bits"=w159, "Buffer"=w151) -> ("Data"=w135:dbl[])  [unwired: 2 in]
            n204 = call "DataBuffer(SubVI).vi"("Bits"=w158, "Buffer"=w150) -> ("Data"=w134:dbl[])  [unwired: 2 in]
            n205 = call "CodeDetection(SubVI).vi"("Code"=w178, "Buff"=w141, "L_sum"=w149) -> ("detect"=w177:bool)
            n206 = call "CodeDetection(SubVI).vi"("Code"=w178, "Buff"=w140, "L_sum"=w148) -> ("detect"=w176:bool)
            n207 = call "CodeDetection(SubVI).vi"("Code"=w178, "Buff"=w139, "L_sum"=w147) -> ("detect"=w175:bool)
            n208 = call "CodeDetection(SubVI).vi"("Code"=w178, "Buff"=w138, "L_sum"=w146) -> ("detect"=w174:bool)
            n209 = call "CodeDetection(SubVI).vi"("Code"=w178, "Buff"=w137, "L_sum"=w145) -> ("detect"=w173:bool)
            n210 = call "CodeDetection(SubVI).vi"("Code"=w178, "Buff"=w136, "L_sum"=w144) -> ("detect"=w172:bool)
            n211 = call "CodeDetection(SubVI).vi"("Code"=w178, "Buff"=w135, "L_sum"=w143) -> ("detect"=w171:bool)
            n212 = call "CodeDetection(SubVI).vi"("Code"=w178, "Buff"=w134, "L_sum"=w142) -> ("detect"=w170:bool)
            n213 = Build Array(w177, w176, w175, w174, w173, w172, w171, w170) -> (w169:bool[])
            n214 = Boolean Array To Number(Boolean array=w169) -> (number=w168:u32)
            n215 = Greater Than 0?(x=w168) -> (x > 0?=w167:bool)
            "Detect" <- w167
            "숫자형 4" <- w166
          }
          n216 = Release Queue(queue=w86, error in (no error)=w85) -> ()  [unwired: 1 in, 3 out]
          n217 = Release Queue(queue=w84, error in (no error)=w83) -> ()  [unwired: 1 in, 3 out]
        }
        frame #2 {
          n218 = local read "Device"() -> (w431:tag)
          n219 = call <vilib>:"DAQmx Reset Device.vi"("device in"=w431) -> ("error out"=w430:errorcluster)  [unwired: 1 in, 13 out]
        }
        frame #3 {
          w436 = dbl[] [-1.0, -1.0, -1.0, -1.0, -1.0, -1.0, -1.0, -1.0]
          w450 = dbl[][] []
          w466 = waveform(dbl) {"t0"=timestamp(0 s since 1904-01-01), "dt"=1.0, "Y"=[]} ("Waveform")
          w439 = "Proc1" ("이름(이름없음)")
          w438 = "Proc0" ("이름(이름없음)")
          w437 = dbl[][] []
          w489 = "SIG0" ("이름(이름없음)")
          w496 = waveform(dbl) {"t0"=timestamp(0 s since 1904-01-01), "dt"=1.0, "Y"=[]} ("Waveform")
          w480 = "SIG1" ("이름(이름없음)")
          w512 = 10123 items=["유한 샘플"=10178, "연속 샘플"=10123, "하드웨어 타이밍에 의한 단일 포인트"=12522] ("sample mode")
          w516 = 10178 items=["유한 샘플"=10178, "연속 샘플"=10123, "하드웨어 타이밍에 의한 단일 포인트"=12522] ("sample mode")
          # "[Post processing]  1. Queue get : Proc0, Proc1 / 2. Threshold estimation with moving average / 3. Peak and valley detection / 4. Demodulation"
          # "[Rx.time]\nTravel time (1km) : 670ms * 2\nDown-link : 210ms\nUp-link : 1024ms\nTotal : Rx.time > 2574ms"
          # "Local variable"
          # "Queue clear"
          # "[Data Acquistion (ADC)]"
          # "Signal generation (Counter) / delaty time : 200ms"
          # "[Signal processing]\n1. Queue get : SIG0\n2. Data type converting : Waveform (DBL) --> Array (DBL)\n3. DDC (Digital to Digital Convering)\n  - DSB modulation : Multiply carrier signal (30kHz)\n  - Decimate : 192kHz sample rate --> 16kHz sample rate\n4. Cross-correlation with down-chirp (4k ~ 0Hz)\n5. Envelope detection (Hilbert transform) & square\n6. Queue put : Proc1"
          # "[Signal processing]\n1. Queue get : SIG0\n2. Data type converting : Waveform (DBL) --> Array (DBL)\n3. DDC (Digital to Digital Convering)\n  - DSB modulation : Multiply carrier signal (30kHz)\n  - Decimate : 192kHz sample rate --> 16kHz sample rate\n4. Cross-correlation with up-chirp (0 ~ 4kHz)\n5. Envelope detection (Hilbert transform) & square\n6. Queue put : Proc0"
          # "[Data Acquistion (ADC)]\n1. Device reset\n2. Creat channel\n3, Set sample clock\n  - Sampling frequency : 192kHz\n  - Number of sample (Chunk size) : 38400\n4. Start task\n5. Data read\n6. Queue put : SIG0, SIG1\n  - Queue data type : Waveform (DBL)"
          n220 = local read "Number of pulse"() -> (w517:i32)
          n221 = local read "Output terminal"() -> (w520:tag)
          n222 = local read "Sampling freuqncy(Hz)"() -> (w448:dbl)
          n223 = local read "Physical channel"() -> (w514:tag)
          n224 = local read "Frequency(Hz)"() -> (w525:dbl)
          n225 = Build Array(w466, w466, w466, w466, w466, w466, w466, w466) -> (w465:waveform(dbl)[])
          n226 = local read "Cycle share"() -> (w524:dbl)
          n227 = local read "Number of sample"() -> (w447:i32)
          n228 = local read "Counter"() -> (w526:tag)
          n229 = Obtain Queue(name (unnamed)="SIG1" ("이름(이름없음)"), element data type=w465) -> (queue out=w462:refnum<queue>, error out=w461:errorcluster)  [unwired: 3 in, 1 out]
          n230 = Obtain Queue(name (unnamed)="Proc1" ("이름(이름없음)"), element data type=w450) -> (queue out=w454:refnum<queue>, error out=w453:errorcluster)  [unwired: 3 in, 1 out]
          n231 = Obtain Queue(name (unnamed)="SIG0" ("이름(이름없음)"), element data type=w465) -> (queue out=w472:refnum<queue>, error out=w471:errorcluster)  [unwired: 3 in, 1 out]
          n232 = Obtain Queue(name (unnamed)="Proc0" ("이름(이름없음)"), element data type=w450) -> (queue out=w460:refnum<queue>, error out=w459:errorcluster)  [unwired: 3 in, 1 out]
          n233 = call-poly <vilib>:"DAQmx Create Virtual Channel.vi"("frequency"=w525, "duty cycle"=w524, "counter"=w526, "error in"=w523) -> ("task out"=w522:refnum<k21>, "error out"=w521:errorcluster)  [unwired: 10 in]
          n234 = call-poly <vilib>:"DAQmx Create Virtual Channel.vi"("physical channels"=w514) -> ("task out"=w513:refnum<k21>, "error out"=w515:errorcluster)  [unwired: 8 in, 5 out]
          n235 = Flush Queue(queue=w472, error in (no error)=w471) -> (queue out=w470:refnum<queue>, error out=w469:errorcluster)  [unwired: 1 out]
          n236 = Flush Queue(queue=w462, error in (no error)=w461) -> (queue out=w464:refnum<queue>, error out=w463:errorcluster)  [unwired: 1 out]
          n237 = Flush Queue(queue=w460, error in (no error)=w459) -> (queue out=w458:refnum<queue>, error out=w457:errorcluster)  [unwired: 1 out]
          n238 = Flush Queue(queue=w454, error in (no error)=w453) -> (queue out=w456:refnum<queue>, error out=w455:errorcluster)  [unwired: 1 out]
          n239 = property class="DAQmx 채널"(reference=w522, error in=w521, "CO.Pulse.Term"=w520) -> (reference out=w519:refnum<k21>, error out=w518:errorcluster)
          n240 = Release Queue(queue=w470, error in (no error)=w469) -> ()  [unwired: 1 in, 3 out]
          n241 = Release Queue(queue=w464, error in (no error)=w463) -> ()  [unwired: 1 in, 3 out]
          n242 = Release Queue(queue=w458, error in (no error)=w457) -> ()  [unwired: 1 in, 3 out]
          n243 = Release Queue(queue=w456, error in (no error)=w455) -> ()  [unwired: 1 in, 3 out]
          n244 = call-poly <vilib>:"DAQmx Timing.vi"("task/channels in"=w513, "sample mode"=w512, "samples per channel"=w447, "rate"=w448, "error in"=w515) -> ("task out"=w511:refnum<k21>, "error out"=w510:errorcluster)  [unwired: 2 in, 7 out]
          n245 = call-poly <vilib>:"DAQmx Timing.vi"("task/channels in"=w519, "sample mode"=w516, "samples per channel"=w517, "error in"=w518) -> ("task out"=w509:refnum<k21>, "error out"=w508:errorcluster)  [unwired: 10 in]
          n246 = flat-sequence {
            tunnel: w511 -> [w823]
            tunnel: w510 -> [w822]
            tunnel: w509 -> [w821]
            tunnel: w508 -> [w820]
            tunnel: [w821] -> w507
            tunnel: [w820] -> w506
            tunnel: [w819] -> w478
            tunnel: [w818] -> w477
            frame #0 {
              n247 = call <vilib>:"DAQmx Start Task.vi"("task/channels in"=w823, "error in"=w822) -> ("task out"=w819:refnum<k21>, "error out"=w818:errorcluster)  [unwired: 12 in]
            }
          }
          n248 = for {
            N: 2 -> [_]
            tunnel: w507 -> [w816]
            tunnel: [w811] -> w504
            tunnel: w506 -> [w817]
            tunnel: [w810] -> w503
            n249 = call <vilib>:"DAQmx Start Task.vi"("task/channels in"=w816, "error in"=w817) -> ("task out"=w815:refnum<k21>, "error out"=w814:errorcluster)  [unwired: 12 in]
            n250 = call <vilib>:"DAQmx Is Task Done.vi"("task/channels in"=w815, "error in"=w814) -> ("task out"=w813:refnum<k21>, "error out"=w812:errorcluster)  [unwired: 11 in, 1 out]
            n251 = Wait (ms)(milliseconds to wait=u32 200 ("대기 시간 (ms)")) -> ()  [unwired: 1 out]
            n252 = call <vilib>:"DAQmx Stop Task.vi"("task/channels in"=w813, "error in"=w812) -> ("task out"=w811:refnum<k21>, "error out"=w810:errorcluster)  [unwired: 12 in]
          }
          n253 = Multiply(x=3.0, y=w448) -> (x*y=w446:dbl)
          n254 = To Double Precision Float(number=w447) -> (double precision float=w445:dbl)
          n255 = Divide(x=w446, y=w445) -> (x/y=w444:dbl)
          n256 = To Long Integer(number=w444) -> (32bit integer=w432:i32)
          n257 = call <vilib>:"DAQmx Clear Task.vi"("task in"=w504, "error in"=w503) -> ()  [unwired: 13 in, 1 out]
          n258 = Build Array(w496, w496, w496, w496, w496, w496, w496, w496) -> (w479:waveform(dbl)[])
          n259 = Obtain Queue(name (unnamed)=w480, element data type=w479) -> (queue out=w498:refnum<queue>, error out=w497:errorcluster)  [unwired: 3 in, 1 out]
          n260 = Obtain Queue(name (unnamed)=w489, element data type=w479) -> (queue out=w495:refnum<queue>, error out=w494:errorcluster)  [unwired: 3 in, 1 out]
          n261 = for {
            N: w432 -> [_]
            tunnel: w478 -> [w808]
            tunnel: w477 -> [w807]
            tunnel: [w806] -> w501
            tunnel: [w805] -> w502
            tunnel: w447 -> [w804]
            tunnel: w498 -> [w803]
            tunnel: w497 -> [w802]
            tunnel: w495 -> [w801]
            tunnel: w494 -> [w800]
            i -> [w798]
            n262 = call-poly <vilib>:"DAQmx Read.vi"("task/channels in"=w808, "number of samples per channel"=w804, "error in"=w807) -> ("task out"=w806:refnum<k21>, "data"=w799:waveform(dbl)[], "error out"=w805:errorcluster)  [unwired: 10 out]
            n263 = Enqueue Element(queue=w801, element=w799, error in (no error)=w800) -> ()  [unwired: 1 in, 3 out]
            n264 = Enqueue Element(queue=w803, element=w799, error in (no error)=w802) -> ()  [unwired: 1 in, 3 out]
            "숫자형 5" <- w798
          }
          n265 = local read "Coefficient_bit1"() -> (w473:dbl[])
          n266 = local read "ThresholdMargin"() -> (w433:dbl)
          n267 = local read "MovingAvrParm"() -> (w434:dbl[])
          n268 = local read "Decimation rate"() -> (w475:i32)
          n269 = local read "Coefficient_bit0"() -> (w474:dbl[])
          n270 = local read "Carrier signal"() -> (w476:dbl[])
          n271 = local read "Target code"() -> (w435:dbl[])
          n272 = call <vilib>:"DAQmx Stop Task.vi"("task/channels in"=w501, "error in"=w502) -> ("task out"=w500:refnum<k21>, "error out"=w499:errorcluster)  [unwired: 12 out]
          n273 = call <vilib>:"DAQmx Clear Task.vi"("task in"=w500, "error in"=w499) -> ()  [unwired: 14 out]
          n274 = Obtain Queue(name (unnamed)=w438, element data type=w437) -> (queue out=w493:refnum<queue>, error out=w492:errorcluster)  [unwired: 3 in, 1 out]
          n275 = Obtain Queue(name (unnamed)=w489, element data type=w479) -> (queue out=w491:refnum<queue>, error out=w490:errorcluster)  [unwired: 3 in, 1 out]
          n276 = for {
            N: w432 -> [_]
            tunnel: w491 -> [w797]
            tunnel: w490 -> [w796]
            tunnel: w493 -> [w795]
            tunnel: w492 -> [w794]
            tunnel: [w793] -> w488
            tunnel: [w792] -> w487
            tunnel: w476 -> [w732]
            tunnel: w475 -> [w731]
            tunnel: w474 -> [w730]
            i -> [w728]
            w742 = TRUE ("averaging")
            w791 = TRUE ("init/cont (init:F)")
            n277 = Dequeue Element(queue=w797, error in (no error)=w796) -> (queue out=w793:refnum<queue>, element=w733:waveform(dbl)[], error out=w792:errorcluster)  [unwired: 2 out]
            n278 = Index Array(array=w733) -> (element #1=w790:waveform(dbl), element #2=w789:waveform(dbl), element #3=w788:waveform(dbl), element #4=w787:waveform(dbl), element #5=w786:waveform(dbl), element #6=w785:waveform(dbl), element #7=w784:waveform(dbl), element #8=w783:waveform(dbl))  [unwired: 8 in]
            n279 = Unbundle By Name(w790) -> ("Y"=w782:dbl[])
            n280 = Unbundle By Name(w789) -> ("Y"=w781:dbl[])
            n281 = Unbundle By Name(w788) -> ("Y"=w780:dbl[])
            n282 = Unbundle By Name(w787) -> ("Y"=w779:dbl[])
            n283 = Unbundle By Name(w786) -> ("Y"=w778:dbl[])
            n284 = Unbundle By Name(w785) -> ("Y"=w777:dbl[])
            n285 = Unbundle By Name(w784) -> ("Y"=w776:dbl[])
            n286 = Unbundle By Name(w783) -> ("Y"=w775:dbl[])
            n287 = Multiply(x=w782, y=w732) -> (x*y=w757:dbl[])
            n288 = Multiply(x=w781, y=w732) -> (x*y=w756:dbl[])
            n289 = Multiply(x=w780, y=w732) -> (x*y=w755:dbl[])
            n290 = Multiply(x=w779, y=w732) -> (x*y=w754:dbl[])
            n291 = Multiply(x=w778, y=w732) -> (x*y=w753:dbl[])
            n292 = Multiply(x=w777, y=w732) -> (x*y=w752:dbl[])
            n293 = Multiply(x=w776, y=w732) -> (x*y=w751:dbl[])
            n294 = Multiply(x=w775, y=w732) -> (x*y=w750:dbl[])
            n295 = call-poly <vilib>:"Decimate (single shot).vi"("averaging"=w742, "decimating factor"=w731, "X"=w752) -> ("Decimated Array"=w745:dbl[])  [unwired: 7 in, 1 out]
            n296 = call-poly <vilib>:"Decimate (single shot).vi"("averaging"=w742, "decimating factor"=w731, "X"=w750) -> ("Decimated Array"=w743:dbl[])  [unwired: 7 in, 1 out]
            n297 = call-poly <vilib>:"Decimate (single shot).vi"("averaging"=w742, "decimating factor"=w731, "X"=w756) -> ("Decimated Array"=w749:dbl[])  [unwired: 7 in, 1 out]
            n298 = call-poly <vilib>:"Decimate (single shot).vi"("averaging"=w742, "decimating factor"=w731, "X"=w754) -> ("Decimated Array"=w747:dbl[])  [unwired: 7 in, 1 out]
            n299 = call-poly <vilib>:"Decimate (single shot).vi"("averaging"=w742, "decimating factor"=w731, "X"=w753) -> ("Decimated Array"=w746:dbl[])  [unwired: 7 in, 1 out]
            n300 = call-poly <vilib>:"Decimate (single shot).vi"("averaging"=w742, "decimating factor"=w731, "X"=w751) -> ("Decimated Array"=w744:dbl[])  [unwired: 7 in, 1 out]
            n301 = call-poly <vilib>:"Decimate (single shot).vi"("averaging"=w742, "decimating factor"=w731, "X"=w757) -> ("Decimated Array"=w758:dbl[])  [unwired: 7 in, 1 out]
            n302 = call-poly <vilib>:"Decimate (single shot).vi"("averaging"=w742, "decimating factor"=w731, "X"=w755) -> ("Decimated Array"=w748:dbl[])  [unwired: 7 in, 1 out]
            n303 = call-poly <vilib>:"FIR Filter.vi"("init/cont (init:F)"=w791, "FIR Coefficients"=w730, "X"=w758) -> ("Filtered X"=w774:dbl[])  [unwired: 1 in, 1 out]
            n304 = call-poly <vilib>:"FIR Filter.vi"("init/cont (init:F)"=w791, "FIR Coefficients"=w730, "X"=w749) -> ("Filtered X"=w773:dbl[])  [unwired: 1 in, 1 out]
            n305 = call-poly <vilib>:"FIR Filter.vi"("init/cont (init:F)"=w791, "FIR Coefficients"=w730, "X"=w748) -> ("Filtered X"=w772:dbl[])  [unwired: 1 in, 1 out]
            n306 = call-poly <vilib>:"FIR Filter.vi"("init/cont (init:F)"=w791, "FIR Coefficients"=w730, "X"=w747) -> ("Filtered X"=w771:dbl[])  [unwired: 1 in, 1 out]
            n307 = call-poly <vilib>:"FIR Filter.vi"("init/cont (init:F)"=w791, "FIR Coefficients"=w730, "X"=w746) -> ("Filtered X"=w770:dbl[])  [unwired: 1 in, 1 out]
            n308 = call-poly <vilib>:"FIR Filter.vi"("init/cont (init:F)"=w791, "FIR Coefficients"=w730, "X"=w745) -> ("Filtered X"=w769:dbl[])  [unwired: 1 in, 1 out]
            n309 = call-poly <vilib>:"FIR Filter.vi"("init/cont (init:F)"=w791, "FIR Coefficients"=w730, "X"=w744) -> ("Filtered X"=w768:dbl[])  [unwired: 1 in, 1 out]
            n310 = call-poly <vilib>:"FIR Filter.vi"("init/cont (init:F)"=w791, "FIR Coefficients"=w730, "X"=w743) -> ("Filtered X"=w767:dbl[])  [unwired: 1 in, 1 out]
            n311 = call "Envelope(SubVI).vi"("x"=w774) -> ("Y"=w766:dbl[])
            n312 = call "Envelope(SubVI).vi"("x"=w773) -> ("Y"=w765:dbl[])
            n313 = call "Envelope(SubVI).vi"("x"=w772) -> ("Y"=w764:dbl[])
            n314 = call "Envelope(SubVI).vi"("x"=w771) -> ("Y"=w763:dbl[])
            n315 = call "Envelope(SubVI).vi"("x"=w770) -> ("Y"=w762:dbl[])
            n316 = call "Envelope(SubVI).vi"("x"=w769) -> ("Y"=w761:dbl[])
            n317 = call "Envelope(SubVI).vi"("x"=w768) -> ("Y"=w760:dbl[])
            n318 = call "Envelope(SubVI).vi"("x"=w767) -> ("Y"=w759:dbl[])
            n319 = Square(x=w766) -> (x^2=w741:dbl[])
            n320 = Square(x=w765) -> (x^2=w740:dbl[])
            n321 = Square(x=w764) -> (x^2=w739:dbl[])
            n322 = Square(x=w763) -> (x^2=w738:dbl[])
            n323 = Square(x=w762) -> (x^2=w737:dbl[])
            n324 = Square(x=w761) -> (x^2=w736:dbl[])
            n325 = Square(x=w760) -> (x^2=w735:dbl[])
            n326 = Square(x=w759) -> (x^2=w734:dbl[])
            n327 = Build Array(w741, w740, w739, w738, w737, w736, w735, w734) -> (w729:dbl[][])
            n328 = Enqueue Element(queue=w795, element=w729, error in (no error)=w794) -> ()  [unwired: 1 in, 3 out]
            "숫자형 6" <- w728
          }
          n329 = Release Queue(queue=w488, error in (no error)=w487) -> ()  [unwired: 1 in, 3 out]
          n330 = Obtain Queue(name (unnamed)=w439, element data type=w437) -> (queue out=w486:refnum<queue>, error out=w485:errorcluster)  [unwired: 3 in, 1 out]
          n331 = Obtain Queue(name (unnamed)=w480, element data type=w479) -> (queue out=w484:refnum<queue>, error out=w483:errorcluster)  [unwired: 3 in, 1 out]
          n332 = for {
            N: w432 -> [_]
            tunnel: w484 -> [w727]
            tunnel: w483 -> [w726]
            tunnel: w486 -> [w725]
            tunnel: w485 -> [w724]
            tunnel: [w723] -> w482
            tunnel: [w722] -> w481
            tunnel: w476 -> [w662]
            tunnel: w475 -> [w661]
            tunnel: w473 -> [w660]
            i -> [w658]
            w672 = TRUE ("averaging")
            w721 = TRUE ("init/cont (init:F)")
            n333 = Dequeue Element(queue=w727, error in (no error)=w726) -> (queue out=w723:refnum<queue>, element=w663:waveform(dbl)[], error out=w722:errorcluster)  [unwired: 2 out]
            n334 = Index Array(array=w663) -> (element #1=w720:waveform(dbl), element #2=w719:waveform(dbl), element #3=w718:waveform(dbl), element #4=w717:waveform(dbl), element #5=w716:waveform(dbl), element #6=w715:waveform(dbl), element #7=w714:waveform(dbl), element #8=w713:waveform(dbl))  [unwired: 8 in]
            n335 = Unbundle By Name(w720) -> ("Y"=w712:dbl[])
            n336 = Unbundle By Name(w719) -> ("Y"=w711:dbl[])
            n337 = Unbundle By Name(w718) -> ("Y"=w710:dbl[])
            n338 = Unbundle By Name(w717) -> ("Y"=w709:dbl[])
            n339 = Unbundle By Name(w716) -> ("Y"=w708:dbl[])
            n340 = Unbundle By Name(w715) -> ("Y"=w707:dbl[])
            n341 = Unbundle By Name(w714) -> ("Y"=w706:dbl[])
            n342 = Unbundle By Name(w713) -> ("Y"=w705:dbl[])
            n343 = Multiply(x=w712, y=w662) -> (x*y=w687:dbl[])
            n344 = Multiply(x=w711, y=w662) -> (x*y=w686:dbl[])
            n345 = Multiply(x=w710, y=w662) -> (x*y=w685:dbl[])
            n346 = Multiply(x=w709, y=w662) -> (x*y=w684:dbl[])
            n347 = Multiply(x=w708, y=w662) -> (x*y=w683:dbl[])
            n348 = Multiply(x=w707, y=w662) -> (x*y=w682:dbl[])
            n349 = Multiply(x=w706, y=w662) -> (x*y=w681:dbl[])
            n350 = Multiply(x=w705, y=w662) -> (x*y=w680:dbl[])
            n351 = call-poly <vilib>:"Decimate (single shot).vi"("averaging"=w672, "decimating factor"=w661, "X"=w682) -> ("Decimated Array"=w675:dbl[])  [unwired: 7 in, 1 out]
            n352 = call-poly <vilib>:"Decimate (single shot).vi"("averaging"=w672, "decimating factor"=w661, "X"=w680) -> ("Decimated Array"=w673:dbl[])  [unwired: 7 in, 1 out]
            n353 = call-poly <vilib>:"Decimate (single shot).vi"("averaging"=w672, "decimating factor"=w661, "X"=w686) -> ("Decimated Array"=w679:dbl[])  [unwired: 7 in, 1 out]
            n354 = call-poly <vilib>:"Decimate (single shot).vi"("averaging"=w672, "decimating factor"=w661, "X"=w684) -> ("Decimated Array"=w677:dbl[])  [unwired: 7 in, 1 out]
            n355 = call-poly <vilib>:"Decimate (single shot).vi"("averaging"=w672, "decimating factor"=w661, "X"=w683) -> ("Decimated Array"=w676:dbl[])  [unwired: 7 in, 1 out]
            n356 = call-poly <vilib>:"Decimate (single shot).vi"("averaging"=w672, "decimating factor"=w661, "X"=w681) -> ("Decimated Array"=w674:dbl[])  [unwired: 7 in, 1 out]
            n357 = call-poly <vilib>:"Decimate (single shot).vi"("averaging"=w672, "decimating factor"=w661, "X"=w687) -> ("Decimated Array"=w688:dbl[])  [unwired: 7 in, 1 out]
            n358 = call-poly <vilib>:"Decimate (single shot).vi"("averaging"=w672, "decimating factor"=w661, "X"=w685) -> ("Decimated Array"=w678:dbl[])  [unwired: 7 in, 1 out]
            n359 = call-poly <vilib>:"FIR Filter.vi"("init/cont (init:F)"=w721, "FIR Coefficients"=w660, "X"=w688) -> ("Filtered X"=w704:dbl[])  [unwired: 1 in, 1 out]
            n360 = call-poly <vilib>:"FIR Filter.vi"("init/cont (init:F)"=w721, "FIR Coefficients"=w660, "X"=w679) -> ("Filtered X"=w703:dbl[])  [unwired: 1 in, 1 out]
            n361 = call-poly <vilib>:"FIR Filter.vi"("init/cont (init:F)"=w721, "FIR Coefficients"=w660, "X"=w678) -> ("Filtered X"=w702:dbl[])  [unwired: 1 in, 1 out]
            n362 = call-poly <vilib>:"FIR Filter.vi"("init/cont (init:F)"=w721, "FIR Coefficients"=w660, "X"=w677) -> ("Filtered X"=w701:dbl[])  [unwired: 1 in, 1 out]
            n363 = call-poly <vilib>:"FIR Filter.vi"("init/cont (init:F)"=w721, "FIR Coefficients"=w660, "X"=w676) -> ("Filtered X"=w700:dbl[])  [unwired: 1 in, 1 out]
            n364 = call-poly <vilib>:"FIR Filter.vi"("init/cont (init:F)"=w721, "FIR Coefficients"=w660, "X"=w675) -> ("Filtered X"=w699:dbl[])  [unwired: 1 in, 1 out]
            n365 = call-poly <vilib>:"FIR Filter.vi"("init/cont (init:F)"=w721, "FIR Coefficients"=w660, "X"=w674) -> ("Filtered X"=w698:dbl[])  [unwired: 1 in, 1 out]
            n366 = call-poly <vilib>:"FIR Filter.vi"("init/cont (init:F)"=w721, "FIR Coefficients"=w660, "X"=w673) -> ("Filtered X"=w697:dbl[])  [unwired: 1 in, 1 out]
            n367 = call "Envelope(SubVI).vi"("x"=w704) -> ("Y"=w696:dbl[])
            n368 = call "Envelope(SubVI).vi"("x"=w703) -> ("Y"=w695:dbl[])
            n369 = call "Envelope(SubVI).vi"("x"=w702) -> ("Y"=w694:dbl[])
            n370 = call "Envelope(SubVI).vi"("x"=w701) -> ("Y"=w693:dbl[])
            n371 = call "Envelope(SubVI).vi"("x"=w700) -> ("Y"=w692:dbl[])
            n372 = call "Envelope(SubVI).vi"("x"=w699) -> ("Y"=w691:dbl[])
            n373 = call "Envelope(SubVI).vi"("x"=w698) -> ("Y"=w690:dbl[])
            n374 = call "Envelope(SubVI).vi"("x"=w697) -> ("Y"=w689:dbl[])
            n375 = Square(x=w696) -> (x^2=w671:dbl[])
            n376 = Square(x=w695) -> (x^2=w670:dbl[])
            n377 = Square(x=w694) -> (x^2=w669:dbl[])
            n378 = Square(x=w693) -> (x^2=w668:dbl[])
            n379 = Square(x=w692) -> (x^2=w667:dbl[])
            n380 = Square(x=w691) -> (x^2=w666:dbl[])
            n381 = Square(x=w690) -> (x^2=w665:dbl[])
            n382 = Square(x=w689) -> (x^2=w664:dbl[])
            n383 = Build Array(w671, w670, w669, w668, w667, w666, w665, w664) -> (w659:dbl[][])
            n384 = Enqueue Element(queue=w725, element=w659, error in (no error)=w724) -> ()  [unwired: 1 in, 3 out]
            "숫자형 7" <- w658
          }
          n385 = Release Queue(queue=w482, error in (no error)=w481) -> ()  [unwired: 1 in, 3 out]
          n386 = Obtain Queue(name (unnamed)=w438, element data type=w437) -> (queue out=w443:refnum<queue>, error out=w442:errorcluster)  [unwired: 3 in, 1 out]
          n387 = Obtain Queue(name (unnamed)=w439, element data type=w437) -> (queue out=w441:refnum<queue>, error out=w440:errorcluster)  [unwired: 3 in, 1 out]
          n388 = for {
            N: w432 -> [_]
            tunnel: w443 -> [w657]
            tunnel: w442 -> [w656]
            tunnel: w441 -> [w655]
            tunnel: w440 -> [w654]
            tunnel: w434 -> [w652]
            tunnel: w433 -> [w616]
            tunnel: [w564] -> _
            tunnel: [w563] -> _
            tunnel: [w562] -> _
            tunnel: [w561] -> _
            tunnel: w435 -> [w560]
            shift-right: [w534] -> _
            shift-left: w436 -> [w550]
            shift-right: [w533] -> _
            shift-left: w436 -> [w549]
            shift-right: [w532] -> _
            shift-left: w436 -> [w548]
            shift-right: [w531] -> _
            shift-left: w436 -> [w547]
            shift-right: [w530] -> _
            shift-left: w436 -> [w546]
            shift-right: [w529] -> _
            shift-left: w436 -> [w545]
            shift-right: [w528] -> _
            shift-left: w436 -> [w544]
            shift-right: [w527] -> _
            shift-left: w436 -> [w543]
            i -> [w559]
            w641 = enum32{"Peaks", "Valleys"}."Valleys" ("peaks/valleys")
            w642 = enum32{"Peaks", "Valleys"}."Peaks" ("peaks/valleys")
            w640 = 5 ("width")
            w651 = TRUE ("init/cont (init:F)")
            n389 = Dequeue Element(queue=w657, error in (no error)=w656) -> (queue out=w564:refnum<queue>, element=w598:dbl[][], error out=w563:errorcluster)  [unwired: 2 out]
            n390 = Dequeue Element(queue=w655, error in (no error)=w654) -> (queue out=w562:refnum<queue>, element=w597:dbl[][], error out=w561:errorcluster)  [unwired: 2 out]
            n391 = Subtract(x=w598, y=w597) -> (x-y=w653:dbl[][])
            n392 = Index Array(array=w653) -> (element #1=w639:dbl[], element #2=w638:dbl[], element #3=w637:dbl[], element #4=w636:dbl[], element #5=w635:dbl[], element #6=w634:dbl[], element #7=w633:dbl[], element #8=w601:dbl[])  [unwired: 16 in]
            n393 = call-poly <vilib>:"FIR Filter.vi"("init/cont (init:F)"=w651, "FIR Coefficients"=w652, "X"=w639) -> ("Filtered X"=w650:dbl[])  [unwired: 1 in, 1 out]
            n394 = call-poly <vilib>:"FIR Filter.vi"("init/cont (init:F)"=w651, "FIR Coefficients"=w652, "X"=w638) -> ("Filtered X"=w649:dbl[])  [unwired: 1 in, 1 out]
            n395 = call-poly <vilib>:"FIR Filter.vi"("init/cont (init:F)"=w651, "FIR Coefficients"=w652, "X"=w637) -> ("Filtered X"=w648:dbl[])  [unwired: 1 in, 1 out]
            n396 = call-poly <vilib>:"FIR Filter.vi"("init/cont (init:F)"=w651, "FIR Coefficients"=w652, "X"=w636) -> ("Filtered X"=w647:dbl[])  [unwired: 1 in, 1 out]
            n397 = call-poly <vilib>:"FIR Filter.vi"("init/cont (init:F)"=w651, "FIR Coefficients"=w652, "X"=w635) -> ("Filtered X"=w646:dbl[])  [unwired: 1 in, 1 out]
            n398 = call-poly <vilib>:"FIR Filter.vi"("init/cont (init:F)"=w651, "FIR Coefficients"=w652, "X"=w634) -> ("Filtered X"=w645:dbl[])  [unwired: 1 in, 1 out]
            n399 = call-poly <vilib>:"FIR Filter.vi"("init/cont (init:F)"=w651, "FIR Coefficients"=w652, "X"=w633) -> ("Filtered X"=w644:dbl[])  [unwired: 1 in, 1 out]
            n400 = call-poly <vilib>:"FIR Filter.vi"("init/cont (init:F)"=w651, "FIR Coefficients"=w652, "X"=w601) -> ("Filtered X"=w643:dbl[])  [unwired: 1 in, 1 out]
            n401 = Array Max & Min(array=w650) -> (max value=w632:dbl, min value=w631:dbl)  [unwired: 2 out]
            n402 = Array Max & Min(array=w649) -> (max value=w630:dbl, min value=w629:dbl)  [unwired: 2 out]
            n403 = Array Max & Min(array=w648) -> (max value=w628:dbl, min value=w627:dbl)  [unwired: 2 out]
            n404 = Array Max & Min(array=w647) -> (max value=w626:dbl, min value=w625:dbl)  [unwired: 2 out]
            n405 = Array Max & Min(array=w646) -> (max value=w624:dbl, min value=w623:dbl)  [unwired: 2 out]
            n406 = Array Max & Min(array=w645) -> (max value=w622:dbl, min value=w621:dbl)  [unwired: 2 out]
            n407 = Array Max & Min(array=w644) -> (max value=w620:dbl, min value=w619:dbl)  [unwired: 2 out]
            n408 = Array Max & Min(array=w643) -> (max value=w618:dbl, min value=w617:dbl)  [unwired: 2 out]
            n409 = call "ThresholdEstimation(SubVI).vi"("Margin"=w616, "최소값"=w629, "최대값"=w630) -> ("N.Th"=w603:dbl, "P.Th"=w614:dbl)
            n410 = call "ThresholdEstimation(SubVI).vi"("Margin"=w616, "최소값"=w627, "최대값"=w628) -> ("N.Th"=w604:dbl, "P.Th"=w613:dbl)
            n411 = call "ThresholdEstimation(SubVI).vi"("Margin"=w616, "최소값"=w625, "최대값"=w626) -> ("N.Th"=w605:dbl, "P.Th"=w612:dbl)
            n412 = call "ThresholdEstimation(SubVI).vi"("Margin"=w616, "최소값"=w623, "최대값"=w624) -> ("N.Th"=w606:dbl, "P.Th"=w611:dbl)
            n413 = call "ThresholdEstimation(SubVI).vi"("Margin"=w616, "최소값"=w631, "최대값"=w632) -> ("N.Th"=w602:dbl, "P.Th"=w615:dbl)
            n414 = call "ThresholdEstimation(SubVI).vi"("Margin"=w616, "최소값"=w621, "최대값"=w622) -> ("N.Th"=w607:dbl, "P.Th"=w610:dbl)
            n415 = call "ThresholdEstimation(SubVI).vi"("Margin"=w616, "최소값"=w619, "최대값"=w620) -> ("N.Th"=w608:dbl, "P.Th"=w609:dbl)
            n416 = call "ThresholdEstimation(SubVI).vi"("Margin"=w616, "최소값"=w617, "최대값"=w618) -> ("N.Th"=w600:dbl, "P.Th"=w599:dbl)
            n417 = call <vilib>:"Peak Detector.vi"("peaks/valleys"=w642, "width"=w640, "threshold"=w615, "X"=w639) -> ("Locations"=w573:dbl[], "# found"=w589:i32)  [unwired: 3 in, 3 out]
            n418 = call <vilib>:"Peak Detector.vi"("peaks/valleys"=w642, "width"=w640, "threshold"=w614, "X"=w638) -> ("Locations"=w574:dbl[], "# found"=w590:i32)  [unwired: 3 in, 3 out]
            n419 = call <vilib>:"Peak Detector.vi"("peaks/valleys"=w642, "width"=w640, "threshold"=w613, "X"=w637) -> ("Locations"=w575:dbl[], "# found"=w591:i32)  [unwired: 3 in, 3 out]
            n420 = call <vilib>:"Peak Detector.vi"("peaks/valleys"=w642, "width"=w640, "threshold"=w612, "X"=w636) -> ("Locations"=w576:dbl[], "# found"=w592:i32)  [unwired: 3 in, 3 out]
            n421 = call <vilib>:"Peak Detector.vi"("peaks/valleys"=w642, "width"=w640, "threshold"=w611, "X"=w635) -> ("Locations"=w577:dbl[], "# found"=w593:i32)  [unwired: 3 in, 3 out]
            n422 = call <vilib>:"Peak Detector.vi"("peaks/valleys"=w642, "width"=w640, "threshold"=w610, "X"=w634) -> ("Locations"=w578:dbl[], "# found"=w594:i32)  [unwired: 3 in, 3 out]
            n423 = call <vilib>:"Peak Detector.vi"("peaks/valleys"=w642, "width"=w640, "threshold"=w609, "X"=w633) -> ("Locations"=w579:dbl[], "# found"=w595:i32)  [unwired: 3 in, 3 out]
            n424 = call <vilib>:"Peak Detector.vi"("peaks/valleys"=w642, "width"=w640, "threshold"=w599, "X"=w601) -> ("Locations"=w580:dbl[], "# found"=w596:i32)  [unwired: 3 in, 3 out]
            n425 = call <vilib>:"Peak Detector.vi"("peaks/valleys"=w641, "width"=w640, "threshold"=w602, "X"=w639) -> ("Locations"=w572:dbl[], "# found"=w588:i32)  [unwired: 3 in, 3 out]
            n426 = call <vilib>:"Peak Detector.vi"("peaks/valleys"=w641, "width"=w640, "threshold"=w603, "X"=w638) -> ("Locations"=w571:dbl[], "# found"=w587:i32)  [unwired: 3 in, 3 out]
            n427 = call <vilib>:"Peak Detector.vi"("peaks/valleys"=w641, "width"=w640, "threshold"=w604, "X"=w637) -> ("Locations"=w570:dbl[], "# found"=w586:i32)  [unwired: 3 in, 3 out]
            n428 = call <vilib>:"Peak Detector.vi"("peaks/valleys"=w641, "width"=w640, "threshold"=w605, "X"=w636) -> ("Locations"=w569:dbl[], "# found"=w585:i32)  [unwired: 3 in, 3 out]
            n429 = call <vilib>:"Peak Detector.vi"("peaks/valleys"=w641, "width"=w640, "threshold"=w606, "X"=w635) -> ("Locations"=w568:dbl[], "# found"=w584:i32)  [unwired: 3 in, 3 out]
            n430 = call <vilib>:"Peak Detector.vi"("peaks/valleys"=w641, "width"=w640, "threshold"=w607, "X"=w634) -> ("Locations"=w567:dbl[], "# found"=w583:i32)  [unwired: 3 in, 3 out]
            n431 = call <vilib>:"Peak Detector.vi"("peaks/valleys"=w641, "width"=w640, "threshold"=w608, "X"=w633) -> ("Locations"=w566:dbl[], "# found"=w582:i32)  [unwired: 3 in, 3 out]
            n432 = call <vilib>:"Peak Detector.vi"("peaks/valleys"=w641, "width"=w640, "threshold"=w600, "X"=w601) -> ("Locations"=w565:dbl[], "# found"=w581:i32)  [unwired: 3 in, 3 out]
            n433 = call "Decision(SubVI).vi"("L_ind0"=w589, "L_ind1"=w588, "Peak_ind0"=w573, "Peak_ind1"=w572) -> ("L_sum"=w542:i32, "Bits"=w558:dbl[])  [unwired: 2 in]
            n434 = call "Decision(SubVI).vi"("L_ind0"=w590, "L_ind1"=w587, "Peak_ind0"=w574, "Peak_ind1"=w571) -> ("L_sum"=w541:i32, "Bits"=w557:dbl[])  [unwired: 2 in]
            n435 = call "Decision(SubVI).vi"("L_ind0"=w591, "L_ind1"=w586, "Peak_ind0"=w575, "Peak_ind1"=w570) -> ("L_sum"=w540:i32, "Bits"=w556:dbl[])  [unwired: 2 in]
            n436 = call "Decision(SubVI).vi"("L_ind0"=w592, "L_ind1"=w585, "Peak_ind0"=w576, "Peak_ind1"=w569) -> ("L_sum"=w539:i32, "Bits"=w555:dbl[])  [unwired: 2 in]
            n437 = call "Decision(SubVI).vi"("L_ind0"=w593, "L_ind1"=w584, "Peak_ind0"=w577, "Peak_ind1"=w568) -> ("L_sum"=w538:i32, "Bits"=w554:dbl[])  [unwired: 2 in]
            n438 = call "Decision(SubVI).vi"("L_ind0"=w594, "L_ind1"=w583, "Peak_ind0"=w578, "Peak_ind1"=w567) -> ("L_sum"=w537:i32, "Bits"=w553:dbl[])  [unwired: 2 in]
            n439 = call "Decision(SubVI).vi"("L_ind0"=w595, "L_ind1"=w582, "Peak_ind0"=w579, "Peak_ind1"=w566) -> ("L_sum"=w536:i32, "Bits"=w552:dbl[])  [unwired: 2 in]
            n440 = call "Decision(SubVI).vi"("L_ind0"=w596, "L_ind1"=w581, "Peak_ind0"=w580, "Peak_ind1"=w565) -> ("L_sum"=w535:i32, "Bits"=w551:dbl[])  [unwired: 2 in]
            n441 = call "DataBuffer(SubVI).vi"("Bits"=w558, "Buffer"=w550) -> ("Data"=w534:dbl[])  [unwired: 2 in]
            n442 = call "DataBuffer(SubVI).vi"("Bits"=w557, "Buffer"=w549) -> ("Data"=w533:dbl[])  [unwired: 2 in]
            n443 = call "DataBuffer(SubVI).vi"("Bits"=w556, "Buffer"=w548) -> ("Data"=w532:dbl[])  [unwired: 2 in]
            n444 = call "DataBuffer(SubVI).vi"("Bits"=w555, "Buffer"=w547) -> ("Data"=w531:dbl[])  [unwired: 2 in]
            n445 = call "DataBuffer(SubVI).vi"("Bits"=w554, "Buffer"=w546) -> ("Data"=w530:dbl[])  [unwired: 2 in]
            n446 = call "DataBuffer(SubVI).vi"("Bits"=w553, "Buffer"=w545) -> ("Data"=w529:dbl[])  [unwired: 2 in]
            n447 = call "DataBuffer(SubVI).vi"("Bits"=w552, "Buffer"=w544) -> ("Data"=w528:dbl[])  [unwired: 2 in]
            n448 = call "DataBuffer(SubVI).vi"("Bits"=w551, "Buffer"=w543) -> ("Data"=w527:dbl[])  [unwired: 2 in]
            n449 = call "CodeDetection(SubVI).vi"("Code"=w560, "Buff"=w534, "L_sum"=w542) -> ()  [unwired: 1 out]
            n450 = call "CodeDetection(SubVI).vi"("Code"=w560, "Buff"=w533, "L_sum"=w541) -> ()  [unwired: 1 out]
            n451 = call "CodeDetection(SubVI).vi"("Code"=w560, "Buff"=w532, "L_sum"=w540) -> ()  [unwired: 1 out]
            n452 = call "CodeDetection(SubVI).vi"("Code"=w560, "Buff"=w531, "L_sum"=w539) -> ()  [unwired: 1 out]
            n453 = call "CodeDetection(SubVI).vi"("Code"=w560, "Buff"=w530, "L_sum"=w538) -> ()  [unwired: 1 out]
            n454 = call "CodeDetection(SubVI).vi"("Code"=w560, "Buff"=w529, "L_sum"=w537) -> ()  [unwired: 1 out]
            n455 = call "CodeDetection(SubVI).vi"("Code"=w560, "Buff"=w528, "L_sum"=w536) -> ()  [unwired: 1 out]
            n456 = call "CodeDetection(SubVI).vi"("Code"=w560, "Buff"=w527, "L_sum"=w535) -> ()  [unwired: 1 out]
            "숫자형 8" <- w559
          }
        }
      }
    }
  }
